vi "ComControlServos.vi"() -> ()   [LabVIEW 2013]
uses:
  <vilib>/Instr/_visa.llb/VISA Configure Serial Port (Instr).vi
panel:
  in  "退出系统":bool
  in  "串口选择":refnum<visa-resource-name>="COM3"
  in  "波特率选择":u16(ring)=9600 items=["9600"=9600, "57600"=57600]
  in  "手臂收回":bool
  out "中间量":string
  in  "清空接收区":bool
  in  "确定按钮":bool
  in  "工作复位":bool
  out "即将要发送角度信息":string
  in  "?":bool
  out "接受区":string
  in  "运行速度":dbl=1.0 min=1.0 max=3.0 step=1.0
  in  "爪子":dbl(slide)=115.0 min=50.0 max=180.0 step=1.0 scale=50.0..180.0 scale format="%_5f"
  in  "手腕":dbl(slide)=90.0 min=0.0 max=180.0 step=1.0 scale=0.0..180.0 scale format="%_5f"
  in  "关节3":dbl(slide)=90.0 min=0.0 max=180.0 step=1.0 scale=0.0..180.0 scale format="%_5f"
  in  "关节2":dbl(slide)=90.0 min=0.0 max=180.0 step=1.0 scale=0.0..180.0 scale format="%_5f"
  in  "关节1":dbl(slide)=90.0 min=0.0 max=180.0 step=1.0 scale=0.0..180.0 scale format="%_5f"
  in  "旋转底座":dbl(slide)=90.0 min=0.0 max=180.0 step=1.0 scale=0.0..180.0 scale format="%_5f"
  # "六自由度机械手姿态调整助手"
  # "By Richard K"
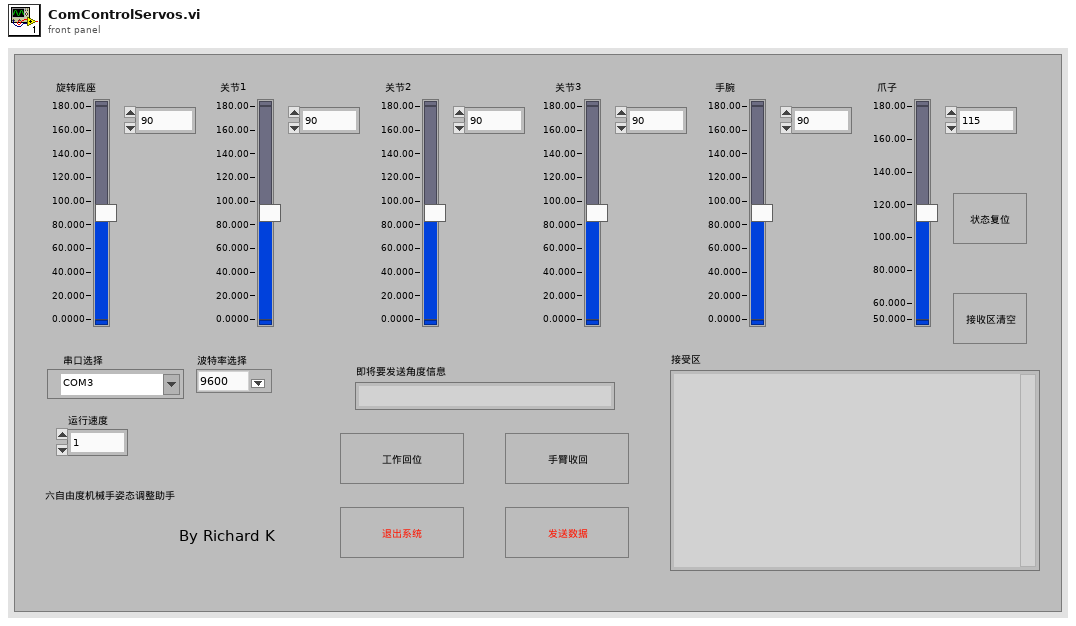
[diagram p1: front panel]
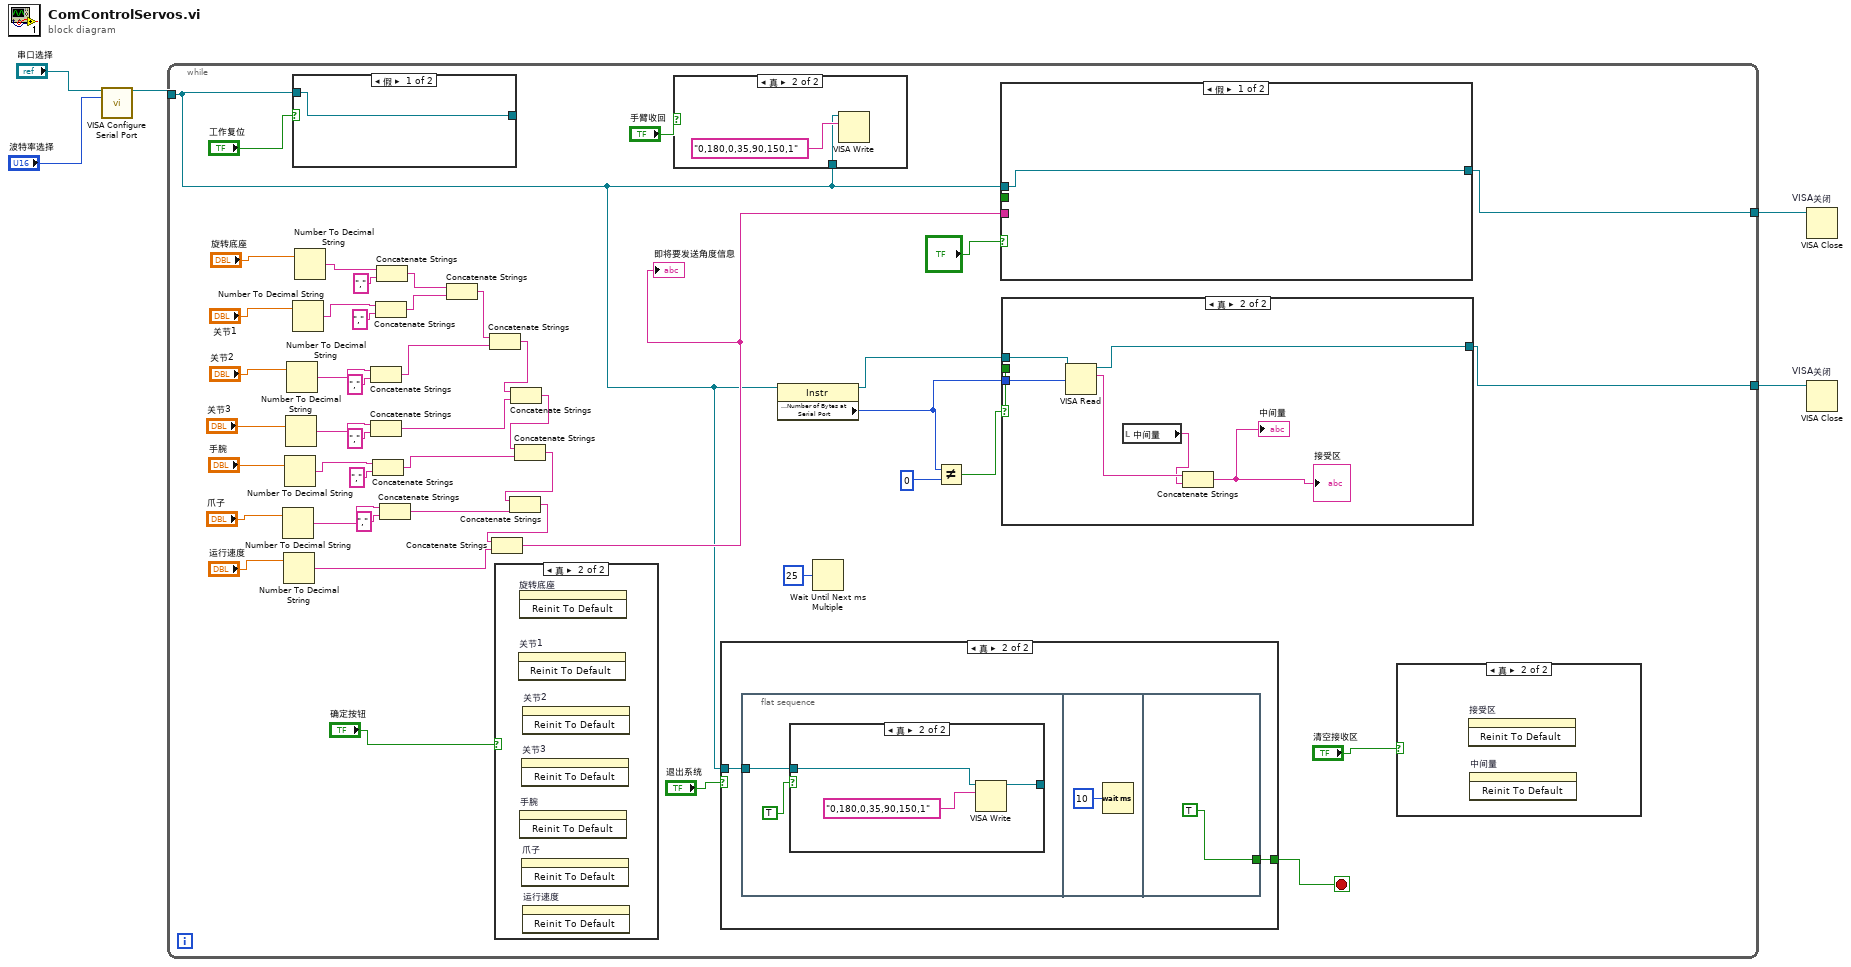
[diagram p0: block diagram]
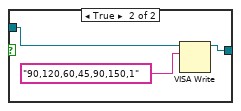
[diagram p7: hidden frame]
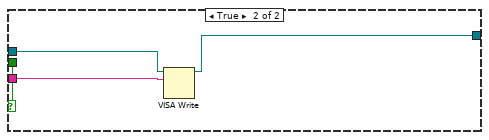
[diagram p9: hidden frame]
diagram:
  n1 = call-poly "VISA Configure Serial Port"("VISA resource name"="串口选择", "baud rate (9600)"="波特率选择") -> ("VISA resource name out"=w3:refnum<visa-resource-name>)  [unwired: 7 in, 6 out]
  n2 = while {
    tunnel: w3 -> [w7]
    tunnel: [w17] -> w5
    tunnel: [w16] -> w4
    stop <- w9 stop-if-true
    n3 = Number To Decimal String(number="爪子") -> (decimal integer string=w26:string)  [unwired: 1 in]
    n4 = Number To Decimal String(number="运行速度") -> (decimal integer string=w23:string)  [unwired: 1 in]
    n5 = Number To Decimal String(number="手腕") -> (decimal integer string=w37:string)  [unwired: 1 in]
    n6 = Number To Decimal String(number="关节3") -> (decimal integer string=w38:string)  [unwired: 1 in]
    n7 = Number To Decimal String(number="关节2") -> (decimal integer string=w39:string)  [unwired: 1 in]
    n8 = case shown="假" "工作复位" {
      tunnel: w7 -> [w64 w66]
      tunnel: [w64 w65] -> _
      frame False {
      }
      frame True {
        n9 = VISA Write(VISA resource name=w66, write buffer="90,120,60,45,90,150,1") -> (VISA resource name out=w65:refnum<visa-resource-name>)  [unwired: 1 in, 2 out]
      }
    }
    n10 = Number To Decimal String(number="关节1") -> (decimal integer string=w40:string)  [unwired: 1 in]
    n11 = Number To Decimal String(number="旋转底座") -> (decimal integer string=w46:string)  [unwired: 1 in]
    n12 = Concatenate Strings(w39, ",") -> (w33:string)
    n13 = Concatenate Strings(w38, ",") -> (w31:string)
    n14 = Concatenate Strings(w37, ",") -> (w29:string)
    n15 = Concatenate Strings(w40, ",") -> (w35:string)
    n16 = Concatenate Strings(w46, ",") -> (w36:string)
    n17 = Concatenate Strings(w26, ",") -> (w25:string)
    n18 = Concatenate Strings(w36, w35) -> (w34:string)
    n19 = Concatenate Strings(w34, w33) -> (w32:string)
    n20 = case shown="真" "确定按钮" {
      frame False {
      }
      frame True {
        n21 = invoke on="关节1" class="Slide (严格)" method="Reinit To Default"() -> ()  [unwired: 3 in, 3 out]
        n22 = invoke on="旋转底座" class="Slide (严格)" method="Reinit To Default"() -> ()  [unwired: 3 in, 3 out]
        n23 = invoke on="手腕" class="Slide (严格)" method="Reinit To Default"() -> ()  [unwired: 3 in, 3 out]
        n24 = invoke on="关节3" class="Slide (严格)" method="Reinit To Default"() -> ()  [unwired: 3 in, 3 out]
        n25 = invoke on="爪子" class="Slide (严格)" method="Reinit To Default"() -> ()  [unwired: 3 in, 3 out]
        n26 = invoke on="关节2" class="Slide (严格)" method="Reinit To Default"() -> ()  [unwired: 3 in, 3 out]
        n27 = invoke on="运行速度" class="DigNum (严格)" method="Reinit To Default"() -> ()  [unwired: 3 in, 3 out]
      }
    }
    n28 = Concatenate Strings(w32, w31) -> (w30:string)
    n29 = Concatenate Strings(w30, w29) -> (w28:string)
    n30 = Concatenate Strings(w28, w25) -> (w24:string)
    n31 = Concatenate Strings(w24, w23) -> (w14:string)
    "即将要发送角度信息" <- w14
    n32 = case shown="真" "手臂收回" {
      tunnel: w7 -> [_ w53]
      frame False {
      }
      frame True {
        n33 = VISA Write(VISA resource name=w53, write buffer="0,180,0,35,90,150,1") -> ()  [unwired: 1 in, 3 out]
      }
    }
    n34 = case shown="真" "退出系统" {
      tunnel: w7 -> [_ w56]
      tunnel: [_ w55] -> w9
      frame False {
      }
      frame True {
        n35 = flat-sequence {
          tunnel: w56 -> [w58]
          tunnel: [TRUE] -> w55
          frame #0 {
            n36 = case shown="真" TRUE {
              tunnel: w58 -> [_ w60]
              tunnel: [_ w59] -> _
              frame False {
              }
              frame True {
                n37 = VISA Write(VISA resource name=w60, write buffer="0,180,0,35,90,150,1") -> (VISA resource name out=w59:refnum<visa-resource-name>)  [unwired: 1 in, 2 out]
              }
            }
          }
          frame #1 {
            n38 = Wait (ms)(milliseconds to wait=u32 10 ("等待时间（毫秒）")) -> ()  [unwired: 1 out]
          }
          frame #2 {
          }
        }
      }
    }
    n39 = property class="Instr"(reference=w7) -> (reference out=w22:refnum<visa-resource-name>, "Serial Settings:Number of Bytes at Serial Port"=w20:u32)  [unwired: 1 in, 1 out]
    n40 = Wait Until Next ms Multiple(millisecond multiple=u32 25 ("毫秒倍数")) -> ()  [unwired: 1 out]
    n41 = Not Equal?(x=w20, y=0) -> (x != y?=w21:bool)
    n42 = case shown="假" "?" {
      selector: "?" -> [_ w80]
      tunnel: [_ w80] -> _
      tunnel: w7 -> [w76 w79]
      tunnel: [w76 w78] -> w17
      tunnel: w14 -> [_ w77]
      frame False {
      }
      frame True {
        n43 = VISA Write(VISA resource name=w79, write buffer=w77) -> (VISA resource name out=w78:refnum<visa-resource-name>)  [unwired: 1 in, 2 out]
      }
    }
    n44 = case shown="真" w21 {
      selector: w21 -> [_ w72]
      tunnel: w22 -> [w68 w75]
      tunnel: [w68 w74] -> w16
      tunnel: w20 -> [_ w73]
      tunnel: [_ w72] -> _
      frame False {
      }
      frame True {
        n45 = VISA Read(VISA resource name=w75, byte count=w73) -> (VISA resource name out=w74:refnum<visa-resource-name>, read buffer=w71:string)  [unwired: 1 in, 2 out]
        n46 = local read "中间量"() -> (w69:string)
        n47 = Concatenate Strings(w71, w69) -> (→"接受区" →"中间量":string)
      }
    }
    n48 = case shown="真" "清空接收区" {
      frame False {
      }
      frame True {
        n49 = invoke on="接受区" class="Str" method="Reinit To Default"() -> ()  [unwired: 3 in, 3 out]
        n50 = invoke on="中间量" class="Str" method="Reinit To Default"() -> ()  [unwired: 3 in, 3 out]
      }
    }
  }
  n51 = VISA Close "VISA关闭"(VISA resource name=w5) -> ()  [unwired: 1 in, 1 out]
  n52 = VISA Close "VISA关闭"(VISA resource name=w4) -> ()  [unwired: 1 in, 1 out]
